vi "WSVCAP SHL Host LL SPI_RFFE Build Socket Mask.vi"(0 "DUT Mask":bool[](array[boolean])) -> (4 "Socket Mask [U16]":u16 format="%04x", 8 "Socket Mask Array":bool[](array[boolean]))   [LabVIEW 2012]
uses:
  Type Defs/WSVCAP SHL DUT Number Enum.ctl
panel:
  in  "DUT":T1
  # "DUT 01"
  # "DUT 02"
  # "DUT 03"
  # "DUT 04"
  # "DUT 05"
  # "DUT 06"
  # "DUT 07"
  # "DUT 08"
  # "DUT 09"
  # "DUT 10"
  # "DUT 11"
  # "DUT 12"
  # "DUT 13"
  # "DUT 14"
  # "DUT 15"
  # "DUT 16"
  # "SKT 01"
  # "SKT 02"
  # "SKT 03"
  # "SKT 04"
  # "SKT 05"
  # "SKT 06"
  # "SKT 07"
  # "SKT 08"
  # "SKT 09"
  # "SKT 10"
  # "SKT 11"
  # "SKT 12"
  # "SKT 13"
  # "SKT 14"
  # "SKT 15"
  # "SKT 16"
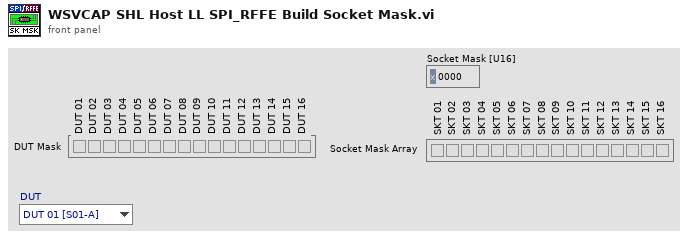
[diagram p1: front panel]
types:
  T1 = typedef "WSVCAP SHL DUT Number Enum.ctl" = enum16{"DUT 01 [S01-A]", "DUT 02 [S02-B]", "DUT 03 [S03-C]", "DUT 04 [S04-D]", "DUT 05 [S05-E]", "DUT 06 [S06-F]", "DUT 07 [S07-G]", "DUT 08 [S08-H]", "DUT 09 [S09-I]", "DUT 10 [S10-J]", "DUT 11 [S11-K]", "DUT 12 [S12-L]", "DUT 13 [S13-M]", "DUT 14 [S14-N]", "DUT 15 [S15-O]", "DUT 16 [S16-P]"}
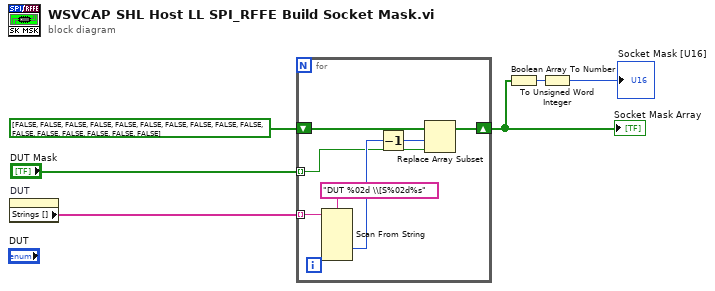
[diagram p0: block diagram]
diagram:
  n1 = property on="DUT" class="Enum (strict)"() -> ("Strings []"=w5:string[])  [unwired: 2 in, 2 out]
  n2 = for {
    tunnel: w5 -> [w13] mode=indexing
    tunnel: "DUT Mask" -> [w8] mode=indexing
    shift-right: [w10] -> w3
    shift-left: bool[] [FALSE, FALSE, FALSE, FALSE, FALSE, FALSE, FALSE, FALSE, FALSE, FALSE, FALSE, FALSE, FALSE, FALSE, FALSE, FALSE] -> [w11]
    n3 = Scan From String(format string="DUT %02d \\[S%02d%s", input string=w13) -> (output 2=w9:i32)  [unwired: 7 in, 3 out]
    n4 = Decrement(x=w9) -> (x-1=w7:i32)
    n5 = Replace Array Subset(array=w11, new element=w8, index=w7) -> (w10:bool[])
  }
  "Socket Mask Array" <- w3
  n6 = Boolean Array To Number(Boolean array=w3) -> (number=w2:u32)
  n7 = To Unsigned Word Integer(number=w2) -> (unsigned 16bit integer=→"Socket Mask [U16]":u16)
